vi "LVClass_CorrectionDataManager ComputeInteractionMatrix.vi"(0 "CorrectionDataManager in":refnum<class "CorrectionDataManager.lvclass">, 7 "HasoSlopes array":refnum<class "HasoSlopes.lvclass">[](array[class]), 11 "error in (no error)":errorcluster) -> (4 "CorrectionDataManager out":refnum<class "CorrectionDataManager.lvclass">, 8 "HasoSlopes array 2":refnum<class "HasoSlopes.lvclass">[](array[class]), 15 "error out":errorcluster)   [LabVIEW 2020, in "CorrectionDataManager.lvclass"]
doc: "Compute interaction matrix from HasoSlopes resulting of the calibration\nperformed.\n\n--------------------------------------------------------------------------------\n\n<B>CorrDataManagerIn </B> : CorrDataManager object.\n<B>CorrDataManagerOut </B> : CorrDataManager object.\n<B>HasoSlopes_array_size </B> : Measured HasoSlopes array size.\n<B>HasoSlopes_array </B> : HasoSlopes measured for each calibration step performed on a valid actuator.\n<B>ErrorIn </B> : Error\n<B>ErrorOut </B> : Error\n\n--------------------------------------------------------------------------------"
uses:
  CorrectionDataManager.lvclass
  HasoSlopes.lvclass
  CorrectionDataManager.lvclass/CorrectionDataManager.ctl
  LVClass_HasoSlopes Read HasoSlopes _ property.vi
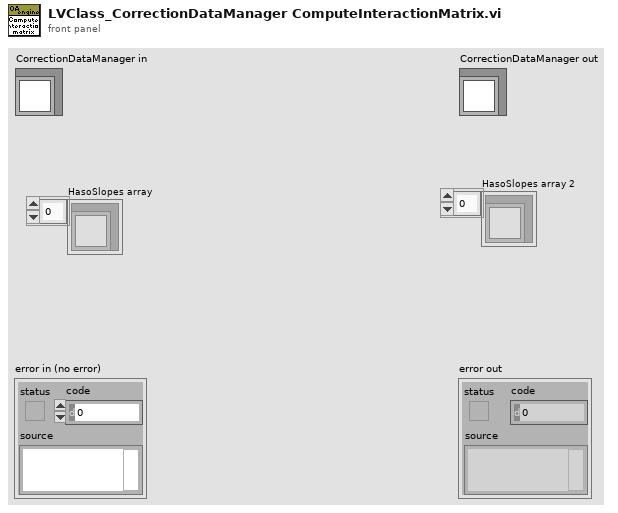
[diagram p1: front panel]
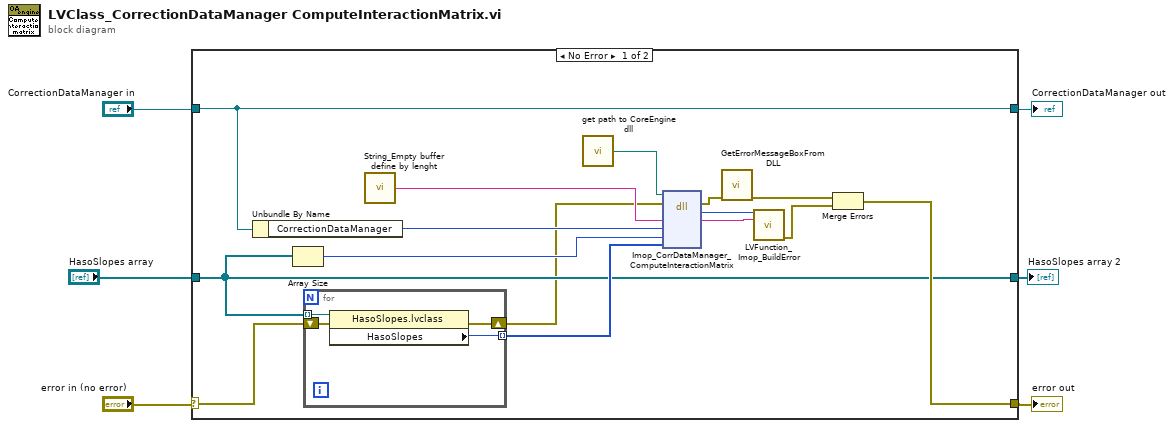
[diagram p0: block diagram]
diagram:
  n1 = case shown="No Error" "error in (no error)" {
    selector: "error in (no error)" -> [w9 w28]
    tunnel: [w14 w28] -> w5
    tunnel: [w12 w27] -> w6
    tunnel: "CorrectionDataManager in" -> [w12 w27]
    tunnel: "HasoSlopes array" -> [w8 w26]
    tunnel: [w8 w26] -> w1
    frame No Error {
      n2 = Unbundle By Name(w12) -> ("CorrectionDataManager"=w13:i32)
      n3 = Array Size(array=w8) -> (size(s)=w10:i32)
      n4 = for {
        tunnel: w8 -> [w24] mode=indexing
        tunnel: [w25] -> w11 mode=indexing
        shift-right: [w22] -> w7
        shift-left: w9 -> [w23]
        n5 = property class="HasoSlopes.lvclass"(reference=w24, error in=w23) -> (error out=w22:errorcluster, "HasoSlopes"=w25:i32)  [unwired: 1 out]
      }
      n6 = call "String_Empty buffer define by lenght.vi"() -> ("Empty buffer"=w19:string)  [unwired: 1 in]
      n7 = call "get path to CoreEngine dll.vi"() -> ("path to c_interface_vc100.dll"=w18:path)  [unwired: 12 in, 3 out]
      n8 = dll-call lib="D:/soft/HASO_v3/SVN_trunk/ImOpCoreEngine4_LV2011/DLLs/c_interface_vc100.dll" fn="Imop_CorrDataManager_ComputeInteractionMatrix"(path in=w18, error in=w7, "message"=w19, "WavefrontCorrection"=w13, "size"=w10, "HasoSlopes array"=w11) -> (error out=w17:errorcluster, "return type"=w21:i32, "message"=w20:string)  [unwired: 4 in, 1 out]
      n9 = call "GetErrorMessageBoxFromDLL.vi"("error IN"=w17) -> ("error OUT"=w16:errorcluster)  [unwired: 10 in]
      n10 = call "LVFunction_Imop_BuildError.vi"("code"=w21, "String to Prepend to source (\"\")"=w20) -> ("error out"=w15:errorcluster)  [unwired: 13 in]
      n11 = Merge Errors(w16, w15) -> (w14:errorcluster)
    }
    frame Error {
    }
  }
  "error out" <- w5
  "CorrectionDataManager out" <- w6
  "HasoSlopes array 2" <- w1
